vi "CSM-TCP-Router(Server).vi"() -> ()   [LabVIEW 2020]
uses:
  <userlib>/_NEVSTOP/Communicable State Machine(CSM)/Utility/_support/Periodic String Filter Level.ctl
  <userlib>/_NEVSTOP/Communicable State Machine(CSM)/Utility/Periodic String Filter Setting.ctl
  931d4ba7-b454-410e-88bd-402e2cce69a9.vi
  e305a403-f40e-4f0c-bbed-de4b6106604b.vi
  <userlib>/_NEVSTOP/Communicable State Machine(CSM)/_Shared/Change Speed Counter.vi
  <userlib>/_NEVSTOP/Communicable State Machine(CSM)/_Shared/Debounced Signal.vi
  931d4ba7-b454-410e-88bd-402e2cce69a9.vi/b09b9099-6be0-413b-8afc-4908471460c3.vi
  <userlib>/_NEVSTOP/Communicable State Machine(CSM)/addons/INI-Static-Variable-Support/_Support/FlagInstance-CSMINIVariable.vi
  <userlib>/_NEVSTOP/Communicable State Machine(CSM)/_Support/ChangeFlag/ChangeFlag-Read.vi
  <userlib>/_NEVSTOP/Communicable State Machine(CSM)/_Support/ChangeFlag/ChangeFlagDB.vi
  <vilib>/Utility/Data Type/Get Type Information.vi
  <userlib>/_NEVSTOP/Communicable State Machine(CSM)/addons/API-String-Arugments-Support/_Support/Data To SingleElementsArray_csm.vi
  <userlib>/_NEVSTOP/Communicable State Machine(CSM)/addons/INI-Static-Variable-Support/_Support/Parse Used Session and Name.vi
  <userlib>/_NEVSTOP/Communicable State Machine(CSM)/addons/API-String-Arugments-Support/_Support/Data To API String Arguments.vi
  <userlib>/_NEVSTOP/Communicable State Machine(CSM)/addons/INI-Static-Variable-Support/_Support/INI-FGV(lvlibp).vi
  <userlib>/_NEVSTOP/Communicable State Machine(CSM)/addons/INI-Static-Variable-Support/_Support/Populate String with INI Variable.vi
  <userlib>/_NEVSTOP/Communicable State Machine(CSM)/addons/API-String-Arugments-Support/_Support/Convert API String Arguments to Data(variant).vi
  <userlib>/_NEVSTOP/Communicable State Machine(CSM)/addons/API-String-Arugments-Support/_Support/SingleElementsArray To Data_csm.vi
  _addons/TCP-Router/_support/Connection Handler Worker.vi
  <vilib>/addons/_JKI.lib/_JKI_lib_TCP_Server.llb/JKI TCP Server.lvclass
  <userlib>/_NEVSTOP/Communicable State Machine(CSM)/Communicable State Machine.lvlib
  _addons/TCP-Router/CSM-TCP-Router.lvlib
  7c227926-344e-407f-80e4-879b129d0d30.vi
  <userlib>/_NEVSTOP/Communicable State Machine(CSM)/_Shared/CSM Shared.lvlib
panel:
  out "LogInQ":i32
  out "State History":string
  out "log handling Speed(#/s)":dbl
  out "LogInQ change(#/s)":dbl
  out "Level":T1
  in  "stop":bool
  out "#Connections":u32
  out "Time Running":dbl[unit] format="%#.0p"
  in  "Disconnect all clients?":bool
  out "Connections Info":T2(array[cluster])
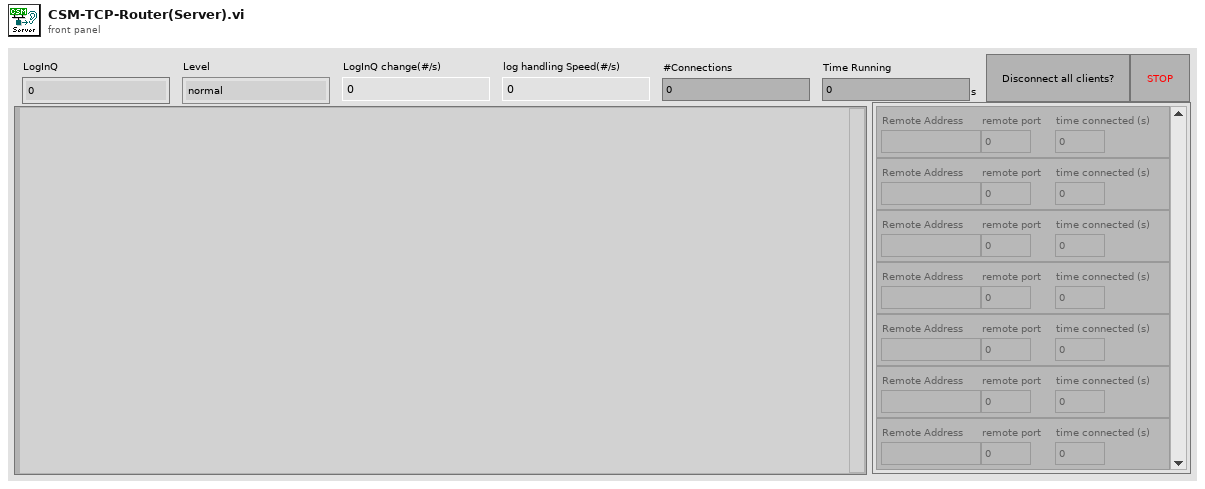
[diagram p1: front panel]
types:
  T1 = typedef "Communicable State Machine.lvlib/Periodic String Filter Level.ctl" = enum16{"normal", "L1", "L2", "L3", "L4"}
  T2 = cluster{"Remote Address":string, "remote port":u16, "time connected (s)":dbl}[]
  T3 = cluster{"Server.Port":u16, "Server.MaxConnections":u32}
  T4 = typedef "JKI TCP Server.lvclass/TCP Server Public Connections Info Cluster.ctl" = cluster{"Remote Address":string, "remote port":u16, "time connected (s)":dbl}
  T5 = typedef "Communicable State Machine.lvlib/Periodic String Filter Setting.ctl" = cluster{"threashold(#/s)":dbl, "Check Peroid(s)":dbl}
  T6 = typedef "Communicable State Machine.lvlib/_CSM_GlobalLog_MSG.ctl" = cluster{"Name (\"\" to Use UUID)":string, "Current State":string, "Arguments":string, "Source Message":T7, "Source Module":string, "Complete(T)/Start(F)":bool, "LogType":T8, "Time Stamp":timestamp}
  T7 = typedef "Communicable State Machine.lvlib/_CSM_Response Source Message.ctl" = cluster{"‘State":string, "’Arguments":string, "’Error":errorcluster}
  T8 = typedef "Communicable State Machine.lvlib/_CSM_GlobalLog_MSG_TYPE.ctl" = enum16{"User Log", "State Change", "Status", "Interrupt", "Register", "Unregister", "Error Log", "Module Created", "Module Destroyed", "Async Message", "No-Rep Async Message", "Sync Message"}
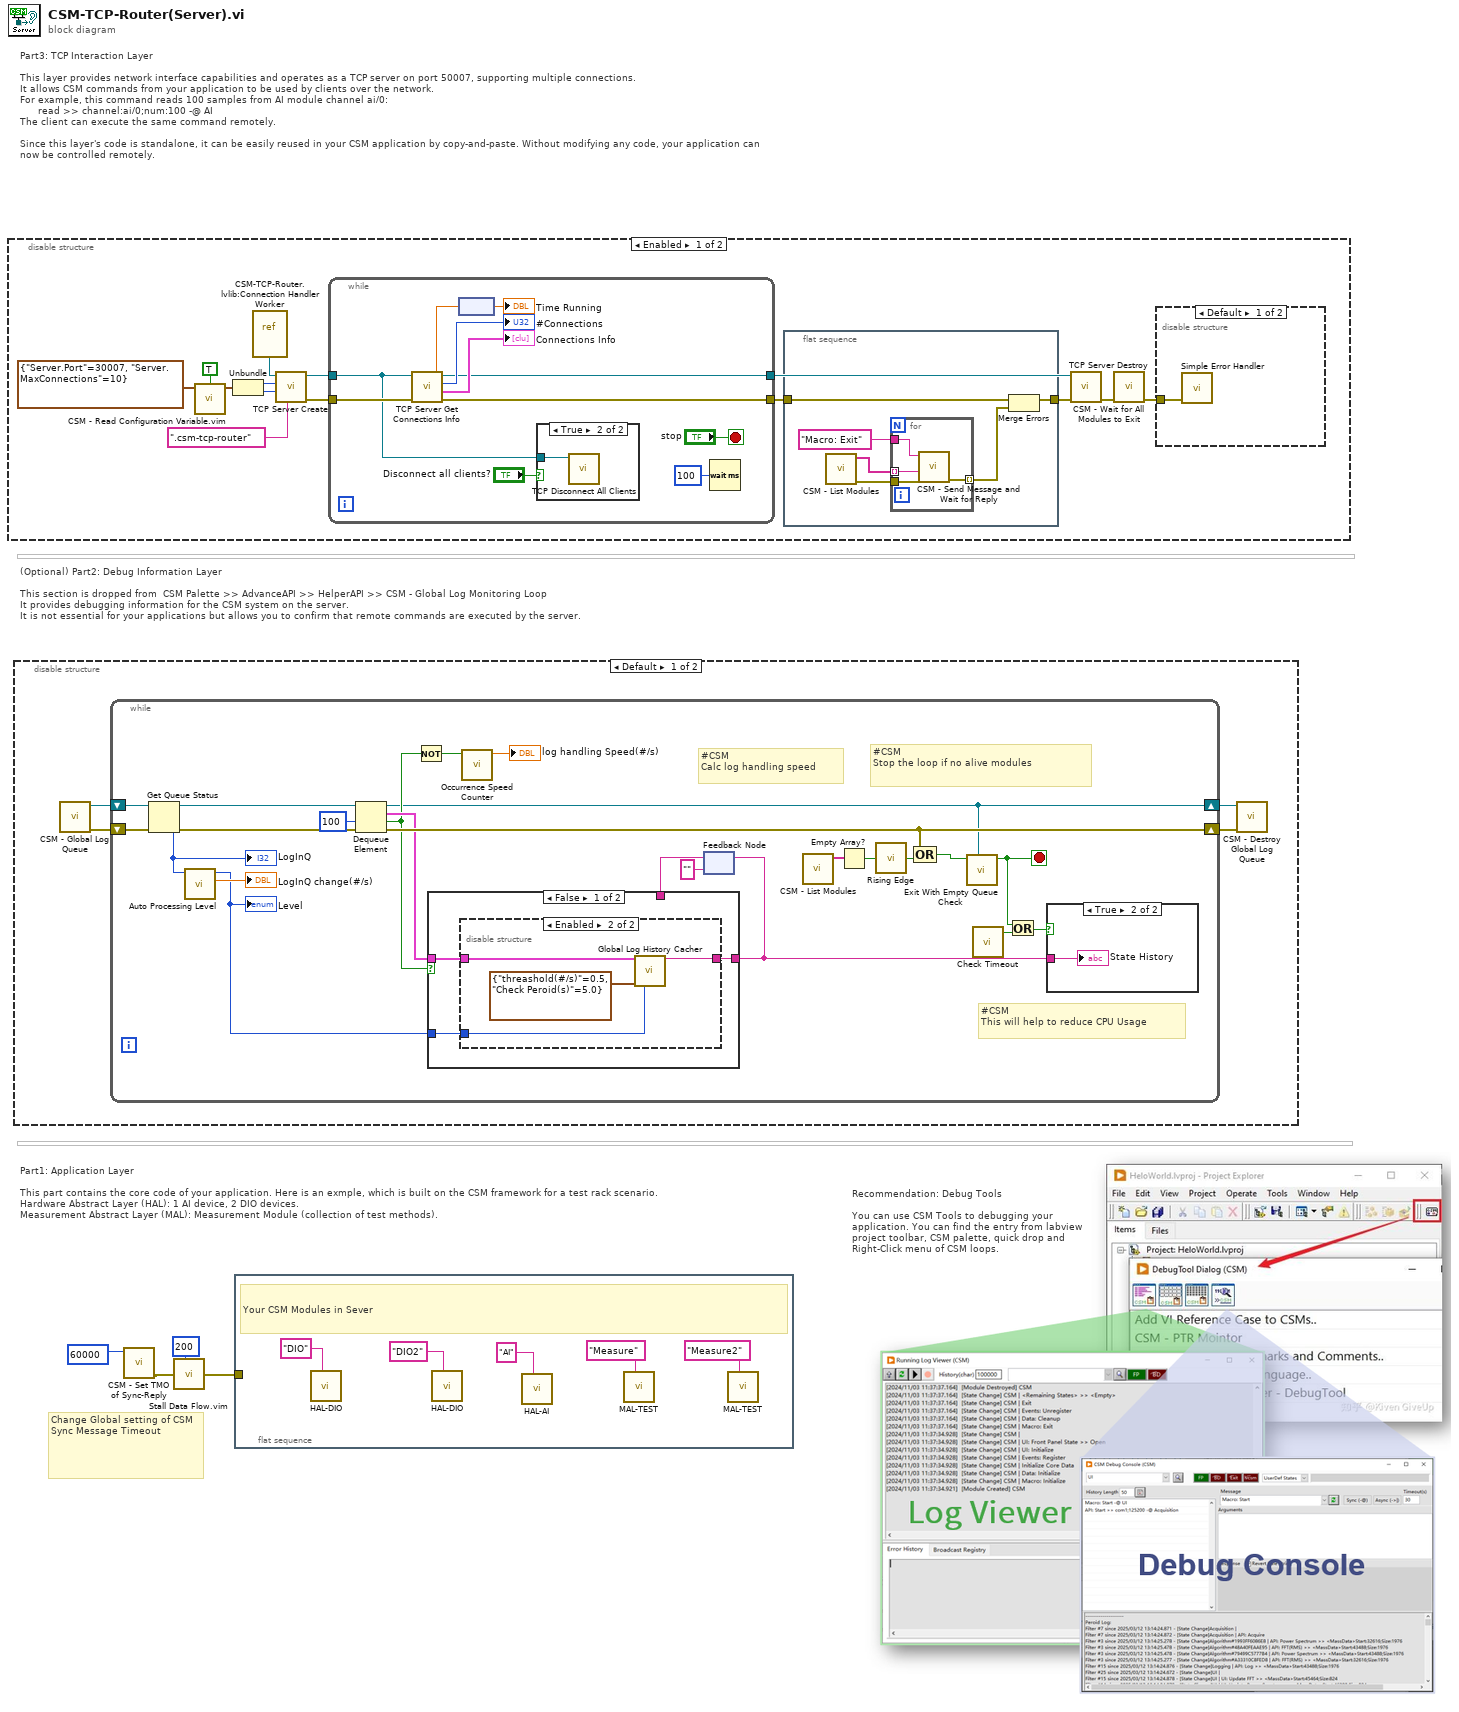
[diagram p0: block diagram]
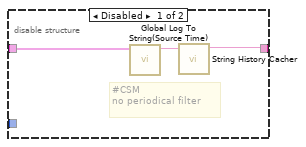
[diagram p2: hidden frame]
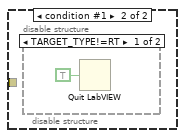
[diagram p7: hidden frame]
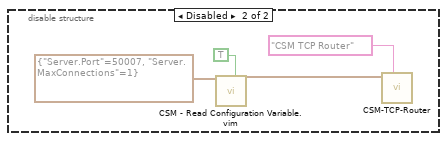
[diagram p9: hidden frame]
diagram:
  # "(Optional) Part2: Debug Information Layer\n\nThis section is dropped from  CSM Palette >> AdvanceAPI >> HelperAPI >> CSM - Global Log Monitoring Loop\nIt provides debugging information for the CSM system on the server. \nIt is not essential for your applications but allows you to confirm that remote commands are executed by the server."
  # "Change Global setting of CSM Sync Message Timeout"
  # "Recommendation: Debug Tools\n\nYou can use CSM Tools to debugging your application. You can find the entry from labview project toolbar, CSM palette, quick drop and Right-Click menu of CSM loops."
  # "Part3: TCP Interaction Layer\n\nThis layer provides network interface capabilities and operates as a TCP server on port 50007, supporting multiple connections. \nIt allows CSM commands from your application to be used by clients over the network. \nFor example, this command reads 100 samples from AI module channel ai/0:\n      read >> channel:ai/0;num:100 -@ AI\nThe client can execute the same command remotely.\n\nSince this layer's code is standalone, it can be easily reused in your CSM application by copy-and-paste. Without modifying any code, your application can now be controlled remotely."
  # "Part1: Application Layer\n\nThis part contains the core code of your application. Here is an exmple, which is built on the CSM framework for a test rack scenario. \nHardware Abstract Layer (HAL): 1 AI device, 2 DIO devices.\nMeasurement Abstract Layer (MAL): Measurement Module (collection of test methods)."
  n1 = disable-structure shown="Enabled" {
    frame Enabled {
      n2 = call "CSM - Read Configuration Variable.vim"("Write If not found? (F)"=TRUE ("Write If not found?(F)"), "Configuration Prototype (Cluster Prefered)"=T3 {"Server.Port"=30007, "Server.MaxConnections"=10}) -> ("Configuration"=w14:T3)  [unwired: 6 in, 1 out]
      n3 = Unbundle(w14) -> ("Server.Port"=w13:u16, "Server.MaxConnections"=w9:u32)
      n4 = vi-ref "CSM-TCP-Router.lvlib:Connection Handler Worker.vi"() -> ("vi reference"=w10:refnum<vi>)
      n5 = call <vilib>:"TCP Server Create.vi"("Additional Data"=".csm-tcp-router", "max connections (0: no limit)"=w9, "port"=w13, "Connection Handler Call-Back VI RefNum"=w10) -> ("error out"=w18:errorcluster, "TCP Server"=w17:refnum<class "JKI TCP Server.lvclass">)  [unwired: 6 in]
      n6 = while {
        tunnel: w18 -> [w34]
        tunnel: w17 -> [w31]
        tunnel: [w33] -> w16
        tunnel: [w32] -> w5
        stop <- "stop" stop-if-true
        n7 = call <vilib>:"TCP Server Get Connections Info.vi"("error in (no error)"=w34, "TCP Server"=w31) -> ("error out"=w32:errorcluster, "Connections Info"=→"Connections Info":T4[], "Number of Connections"=→"#Connections":u32, "TCP Server out"=w33:refnum<class "JKI TCP Server.lvclass">, "time running (s)"=w37:dbl)  [unwired: 5 in]
        n8 = node(w37) -> (→"Time Running":dbl[unit])
        n9 = case shown="True" "Disconnect all clients?" {
          tunnel: w31 -> [_ w40]
          frame False {
          }
          frame True {
            n10 = call <vilib>:"TCP Disconnect All Clients.vi"("TCP Server"=w40) -> ()  [unwired: 9 in, 2 out]
          }
        }
        n11 = Wait (ms)(milliseconds to wait=u32 100) -> ()  [unwired: 1 out]
      }
      n12 = flat-sequence {
        tunnel: [w24] -> w12
        tunnel: w5 -> [w19]
        frame #0 {
          n13 = call <userlib>:"CSM - List Modules.vi"() -> ("error out"=w23:errorcluster, "Module Names"=w22:string[])  [unwired: 10 in]
          n14 = for {
            tunnel: w23 -> [w28]
            tunnel: w22 -> [w27] mode=indexing
            tunnel: "Macro: Exit" ("State") -> [w26]
            tunnel: [w25] -> w20 mode=indexing
            n15 = call <userlib>:"CSM - Send Message and Wait for Reply.vi"("Error In (No Error)"=w28, "Target Module"=w27, "State"=w26) -> ("error out"=w25:errorcluster)  [unwired: 6 in, 2 out]
          }
          n16 = Merge Errors(w19, w20) -> (w24:errorcluster)
        }
      }
      n17 = call <vilib>:"TCP Server Destroy.vi"("error in (no error)"=w12, "TCP Server"=w16) -> ("error out"=w8:errorcluster)  [unwired: 9 in]
      n18 = call <userlib>:"CSM - Wait for All Modules to Exit.vi"("Error In"=w8) -> ("error out"=w7:errorcluster)  [unwired: 8 in, 2 out]
      n19 = disable-structure shown="Default" {
        disable-tunnel: w7 -> [w41 _]
        frame condition #0 (active) {
          n20 = call <vilib>:"Simple Error Handler.vi"("error in (no error)"=w41) -> ()  [unwired: 4 in, 5 out]
        }
        frame condition #1 {
          n21 = disable-structure shown="TARGET_TYPE!=RT" {
            frame condition #0 (active) {
              n22 = Quit LabVIEW(quit? (T)=TRUE) -> ()
            }
            frame condition #1 {
            }
          }
        }
      }
    }
    frame Disabled {
      n23 = call "CSM - Read Configuration Variable.vim"("Write If not found? (F)"=TRUE ("Write If not found?(F)"), "Configuration Prototype (Cluster Prefered)"=T3 {"Server.Port"=50007, "Server.MaxConnections"=1}) -> ("Configuration"=w43:T3)  [unwired: 6 in, 1 out]
      n24 = call "CSM-TCP-Router.vi"("Name(\"\" to use uuid)"="CSM TCP Router" ("Name(\"\" to use uuid)"), "ServerInfo"=w43) -> ()  [unwired: 10 in]
    }
  }
  n25 = disable-structure shown="Default" {
    frame condition #0 (active) {
      n26 = call <userlib>:"CSM - Global Log Queue.vi"() -> ("error out"=w49:errorcluster, "Global Log Queue"=w47:refnum<queue>)  [unwired: 10 in]
      n27 = while {
        shift-right: [w73] -> w50
        shift-left: w49 -> [w70]
        shift-right: [w57] -> w48
        shift-left: w47 -> [w74]
        stop <- w51 stop-if-true
        # "#CSM\nCalc log handling speed"
        # "#CSM\nStop the loop if no alive modules"
        # "#CSM\nThis will help to reduce CPU Usage"
        n28 = Get Queue Status(queue=w74, error in (no error)=w70) -> (queue out=w72:refnum<queue>, error out=w71:errorcluster, # elements in queue=w53:i32)  [unwired: 1 in, 5 out]
        "LogInQ" <- w53
        n29 = call <userlib>:"Auto Processing Level.vi"("#Left In Q"=w53) -> ("LogInQ Changing Speed (#/s)"=→"LogInQ change(#/s)":dbl, "Level"=w52:T1)  [unwired: 8 in, 1 out]
        "Level" <- w52
        n30 = Dequeue Element(queue=w72, timeout in ms (-1)=100, error in (no error)=w71) -> (queue out=w57:refnum<queue>, element=w69:T6, timed out?=w59:bool, error out=w73:errorcluster)
        n31 = Not(x=w59) -> (.not. x?=w58:bool)
        n32 = call <userlib>:"Occurrence Speed Counter.vi"("Occured? (T)"=w58) -> ("Speed (#/s)"=→"log handling Speed(#/s)":dbl)  [unwired: 8 in, 2 out]
        n33 = feedback #1("" ("String Cache")) -> (w65:string)
        n34 = case shown="False" w59 {
          tunnel: w69 -> [w77 _]
          tunnel: [w76 w85] -> w66
          tunnel: w65 -> [_ w85]
          tunnel: w52 -> [w75 _]
          frame False {
            n35 = disable-structure shown="Enabled" {
              disable-tunnel: w77 -> [w80 w83]
              disable-tunnel: [w78 w84] -> w76
              disable-tunnel: w75 -> [_ w82]
              frame Disabled {
                # "#CSM \nno periodical filter"
                n36 = call <userlib>:"Global Log To String(Source Time).vi"("Log"=w80) -> ("Log String"=w79:string)  [unwired: 9 in]
                n37 = call <userlib>:"String History Cacher.vi"("String"=w79) -> ("String Cache"=w78:string)  [unwired: 10 in]
              }
              frame Enabled {
                n38 = call <userlib>:"Global Log History Cacher.vi"("Global Log Data"=w83, "Settings"=T5 {"threashold(#/s)"=0.5, "Check Peroid(s)"=5.0}, "Level (Normal)"=w82) -> ("String Cache"=w84:string)  [unwired: 12 in]
              }
            }
          }
          frame True {
          }
        }
        n39 = feedback-in #1(w66) -> ()
        n40 = call <userlib>:"CSM - List Modules.vi"() -> ("Module Names"=w64:string[])  [unwired: 10 in, 1 out]
        n41 = Empty Array?(array=w64) -> (empty?=w63:bool)
        n42 = call <userlib>:"Rising Edge.vi"("Signal"=w63) -> ("Rising Edge"=w62:bool)
        n43 = Compound Arithmetic op=OR(w73, w62) -> (w55:bool)
        n44 = call <userlib>:"Exit With Empty Queue Check.vi"("Queue"=w57, "Stop"=w55) -> ("Exit"=w51:bool)  [unwired: 8 in, 1 out]
        n45 = call <userlib>:"Check Timeout.vi"() -> ("Timeout"=w67:bool)  [unwired: 8 in]
        n46 = Or(x=w51, y=w67) -> (x .or. y?=w56:bool)
        n47 = case shown="True" w56 {
          tunnel: w66 -> [_ w86]
          frame False {
          }
          frame True {
            "State History" <- w86
          }
        }
      }
      n48 = call <userlib>:"CSM - Destroy Global Log Queue.vi"("Error In"=w50, "Global Log Queue"=w48) -> ()  [unwired: 9 in, 1 out]
    }
    frame condition #1 {
    }
  }
  n49 = call <userlib>:"CSM - Set TMO of Sync-Reply.vi"("TMO For Sync-Rep (ms) In"=60000 ("TMO for Sync-Rep(ms) In")) -> ("error out"=w1:errorcluster)  [unwired: 9 in, 1 out]
  n50 = call "Stall Data Flow.vim"("value in"=w1, "milliseconds to wait"=u32 200) -> ("value out"=w4:errorcluster)  [unwired: 1 out]
  n51 = flat-sequence {
    tunnel: w4 -> [_]
    frame #0 {
      # "Your CSM Modules in Sever"
      n52 = call "HAL-DIO.vi"("Name(\"\" to use uuid)"="DIO" ("Name(\"\" to use uuid)")) -> ()  [unwired: 11 in]
      n53 = call "HAL-DIO.vi"("Name(\"\" to use uuid)"="DIO2" ("Name(\"\" to use uuid)")) -> ()  [unwired: 11 in]
      n54 = call "HAL-AI.vi"("Name(\"\" to use uuid)"="AI" ("Name(\"\" to use uuid)")) -> ()  [unwired: 11 in]
      n55 = call "MAL-TEST.vi"("Name(\"\" to use uuid)"="Measure" ("Name(\"\" to use uuid)")) -> ()  [unwired: 11 in]
      n56 = call "MAL-TEST.vi"("Name(\"\" to use uuid)"="Measure2" ("Name(\"\" to use uuid)")) -> ()  [unwired: 11 in]
    }
  }
